vi "RT Main.vi"() -> ()   [LabVIEW 2019]
doc: "The myRIO Custom FPGA Project template acquires button data from the onboard button and displays the button value on a Boolean indicator. The SYS.RDY indicator shows the FPGA status."
uses:
  <vilib>/Platform/TimedLoop/XDataNode/timing_clust.ctl
  <vilib>/Platform/TimedLoop/XDataNode/nitl_modes.ctl
  <vilib>/Platform/TimedLoop/XDataNode/wakeup.ctl
  <vilib>/myRIO/Instrument Drivers/Onboard IO/DIO/typedefs/DIO Reference.ctl
  <vilib>/myRIO/Common/Instrument Driver Framework/Utilities/typedefs/myRIO Generic Hardware Reference.ctl
  <vilib>/myRIO/Common/Instrument Driver Framework/Utilities/typedefs/Hardware Version Enum.ctl
  <vilib>/myRIO/Common/Instrument Driver Framework/Utilities/typedefs/myRIO v1.0 Reference.ctl
  <vilib>/myRIO/Common/Instrument Driver Framework/Utilities/typedefs/Generic FPGA Reference.ctl
  <vilib>/myRIO/Common/Instrument Driver Framework/myRIO v1.0/DIO/typedefs/DIO Channels List.ctl
  <vilib>/myRIO/Common/Instrument Driver Framework/myRIO v1.0/DIO/typedefs/DIO Channels Enum.ctl
  <vilib>/userDefined/High Color/nirio_resource_hc.ctl
  <vilib>/myRIO/Common/Instrument Driver Framework/myRIO v1.0/Encoder/typedefs/Encoder Signal Mode.ctl
  <vilib>/myRIO/Instrument Drivers/Onboard IO/Encoder/typedefs/Encoder Reference.ctl
  <vilib>/myRIO/Common/Instrument Driver Framework/myRIO v1.0/Encoder/typedefs/Encoder Channels Enum.ctl
  <vilib>/myRIO/Common/Instrument Driver Framework/myRIO v1.0/Encoder/typedefs/Encoder Configuration v1.0.ctl
  <vilib>/myRIO/Instrument Drivers/Onboard IO/AO/typedefs/AO Reference.ctl
  <vilib>/myRIO/Common/Instrument Driver Framework/myRIO v1.0/AO/typedefs/AO Channels List.ctl
  <vilib>/myRIO/Common/Instrument Driver Framework/myRIO v1.0/AO/typedefs/AO Channels Enum.ctl
  <vilib>/myRIO/Common/Instrument Driver Framework/Utilities/typedefs/Analog Scaling Constants List.ctl
  <vilib>/myRIO/Common/Instrument Driver Framework/Utilities/typedefs/Analog Scaling Constants.ctl
  <vilib>/myRIO/Common/Instrument Driver Framework/Utilities/vis/Is FPGA Ref Available.vi
  <vilib>/myRIO/Common/Instrument Driver Framework/myRIO v1.0/DIO/vis/myRIO v1.1 Open DIO.vi
  <vilib>/myRIO/Instrument Drivers/Onboard IO/DIO/vis/Read.vi
  <vilib>/myRIO/Instrument Drivers/Onboard IO/DIO/vis/Write.vi
  <vilib>/myRIO/Common/Instrument Driver Framework/myRIO v1.0/Encoder/vis/myRIO v1.1 Open Encoder.vi
  <vilib>/myRIO/Instrument Drivers/Onboard IO/Encoder/vis/Read.vi
  <vilib>/myRIO/Common/Instrument Driver Framework/myRIO v1.0/AO/vis/myRIO v1.1 Open AO.vi
  <vilib>/myRIO/Instrument Drivers/Onboard IO/AO/vis/Write.vi
  <vilib>/myRIO/Common/Instrument Driver Framework/Utilities/vis/Validate Channels.vi
  <vilib>/myRIO/Common/Instrument Driver Framework/myRIO v1.0/DIO/vis/myRIO v1.0 Reserve DIO.vi
  <vilib>/myRIO/Common/Instrument Driver Framework/myRIO v1.0/Encoder/vis/myRIO v1.0 Reserve Encoder.vi
  <vilib>/myRIO/Common/Instrument Driver Framework/myRIO v1.0/AO/vis/myRIO v1.0 Reserve AO.vi
  <vilib>/myRIO/Common/Instrument Driver Framework/myRIO v1.0/Resource Manager/vis/myRIO v1.0 Reserve Channel List.vi
  <vilib>/myRIO/Common/Instrument Driver Framework/myRIO v1.0/DIO/vis/myRIO v1.0 Build MUX Configuration DIO.vi
  <vilib>/myRIO/Common/Instrument Driver Framework/myRIO v1.0/Encoder/vis/myRIO v1.0 Build MUX Configuration Encoder.vi
  <vilib>/myRIO/Common/Instrument Driver Framework/myRIO v1.0/AO/vis/myRIO v1.0 Build MUX Configuration AO.vi
  <vilib>/myRIO/Common/Instrument Driver Framework/myRIO v1.0/Resource Manager/vis/myRIO v1.0 Reserve Channel.vi
  <vilib>/myRIO/Common/Instrument Driver Framework/myRIO v1.0/Resource Manager/vis/myRIO v1.0 Unreserve Channel.vi
  <vilib>/myRIO/Common/Instrument Driver Framework/myRIO v1.0/Resource Manager/vis/myRIO v1.0 Create Configuration List.vi
  <vilib>/myRIO/Common/Instrument Driver Framework/myRIO v1.0/Resource Manager/vis/myRIO v1.0 Build Mutex Name.vi
  <vilib>/FPGAPlugInAG/myRIO-1900/niLvFpga_Open_myRIO-1900.vi
  <vilib>/rvi/interface/common/dynamic/niFpgaDynamicAddResources.vi
  <vilib>/myRIO/Common/Instrument Driver Framework/Utilities/vis/FPGA Ref Manager.vi
  <vilib>/Utility/error.llb/Error Cluster From Error Code.vi
  <vilib>/myRIO/Common/Instrument Driver Framework/Utilities/vis/Ref Counter.vi
  <vilib>/Utility/VariantDataType/GetNumericInfo.vi
  <vilib>/myRIO/Common/Instrument Driver Framework/myRIO v1.0/myRIO v1.1 Open.vi
  <vilib>/myRIO/Common/Instrument Driver Framework/Utilities/vis/IO Manager.vi
  <vilib>/myRIO/Common/Instrument Driver Framework/Utilities/vis/Configuration Manager.vi
  <vilib>/myRIO/Common/Instrument Driver Framework/myRIO v1.0/Resource Manager/vis/myRIO v1.0 Configure IO.vi
  <vilib>/myRIO/Common/Instrument Driver Framework/myRIO v1.0/myRIO v1.0 Close.vi
  <vilib>/myRIO/Common/Instrument Driver Framework/myRIO v1.0/DIO/vis/myRIO v1.0 Read DIO.vi
  <vilib>/myRIO/Common/Instrument Driver Framework/myRIO v1.0/DIO/vis/myRIO v1.0 Write DIO.vi
  <vilib>/myRIO/Common/Instrument Driver Framework/myRIO v1.0/Encoder/vis/myRIO v1.0 Configure Encoder.vi
  <vilib>/myRIO/Common/Instrument Driver Framework/myRIO v1.0/Encoder/vis/myRIO v1.0 Read Encoder.vi
  <vilib>/myRIO/Common/Instrument Driver Framework/myRIO v1.0/AO/vis/myRIO v1.0 Get Scaling Constants AO.vi
  <vilib>/myRIO/Common/Instrument Driver Framework/myRIO v1.0/AO/vis/myRIO v1.0 Write AO.vi
  <vilib>/FPGAPlugInAG/Dynamic/niLvFpga_Close_Dynamic.vi
  <vilib>/rvi/interface/nirviOpenFPGA/nirviOpenFPGA.xnode
  FPGA Bitfiles/hapticdevice2dof_FPGATarget_FPGAMainDefault_0mKZiwDuvEs.lvbitx
  FPGA Main Default.vi
  <vilib>/Platform/TimedLoop/XDataNode/XDataNode.xnode
  <vilib>/myRIO/Express VI/Onboard Devices/Button/Button Express VI.xnode
  <vilib>/myRIO/Instrument Drivers/Onboard IO/DIO/vis/myRIO DIO Open.xnode
  <vilib>/myRIO/Express VI/Onboard IO/DI/DI Express VI.xnode
  <vilib>/myRIO/Express VI/Onboard Devices/LED/LED Express VI.xnode
  <vilib>/myRIO/Express VI/Onboard IO/Encoder/Encoder Express VI.xnode
  <vilib>/myRIO/Instrument Drivers/Onboard IO/Encoder/vis/myRIO Encoder Open.xnode
  <vilib>/myRIO/Common/Instrument Driver Framework/myRIO v1.0/Encoder/typedefs/Encoder Count Direction Enum.ctl
  <vilib>/myRIO/Express VI/Onboard IO/DO/DO Express VI.xnode
  <vilib>/myRIO/Express VI/Onboard IO/AO/AO Express VI.xnode
  <vilib>/myRIO/Instrument Drivers/Onboard IO/AO/vis/myRIO AO Open.xnode
  <vilib>/rvi/interface/nirviCloseFPGA/nirviCloseFPGA.xnode
  <vilib>/myRIO/Instrument Drivers/Utilities/Utilities.lvlib
  <vilib>/Platform/TimedLoop/XDataNode/XDNodeRunTimeDep.lvlib
  <vilib>/myRIO/Instrument Drivers/Onboard IO/Encoder/Encoder.lvlib
  <vilib>/myRIO/Instrument Drivers/Onboard IO/DIO/DIO.lvlib
  <vilib>/myRIO/Instrument Drivers/Onboard IO/AO/AO.lvlib
panel:
  in  "Ctrl Hz":i64=1000
  in  "TX Hz":i64=1000
  in  "RX Hz":i64=1000
  out "Encoder Reset":bool
  out "Controller\nFinished Late":bool
  out "UDP Read\nFinished Late":bool
  out "UDP Write\nFinished Late":bool
  out "Index":bool
  in  "Current Limit":dbl=1.0
  out "UDP":bool
  out "y_0":dbl
  out "x_0":dbl
  out "STOP":bool
  out "Status":i32
  out "F_y":dbl
  out "F_x":dbl
  in  "?":bool
  in  "Direction A":bool
  in  "Direction B":bool
  in  "Current A":dbl(slide) scale=0.0..10.0
  in  "Current B":dbl(slide) scale=0.0..10.0
  in  "switch":bool=TRUE
  in  "Enable":bool=TRUE
  out "I_0":dbl format="%#.2g"
  out "I_1":dbl format="%#.2g"
  out "f_x":dbl
  out "f_y":dbl
  out "x":dbl format="%#.2g"
  out "y":dbl format="%#.2g"
  out "XY 그래프":cluster{dbl[], dbl[]}(graph)={[-0.04564152437153268], [-0.14073615837554598]}
  out "y_dot":dbl
  out "x_dot":dbl
  in  "Stiff":dbl=1.0
  in  "Damp":dbl
  out "Counter A":i32
  out "Counter B":i32
  out "ENC A":ext
  out "ENC B":ext
  out "count":ext format="%-#.3g"
  out "miss":u32
  out "error out":errorcluster
  # "Manual Control"
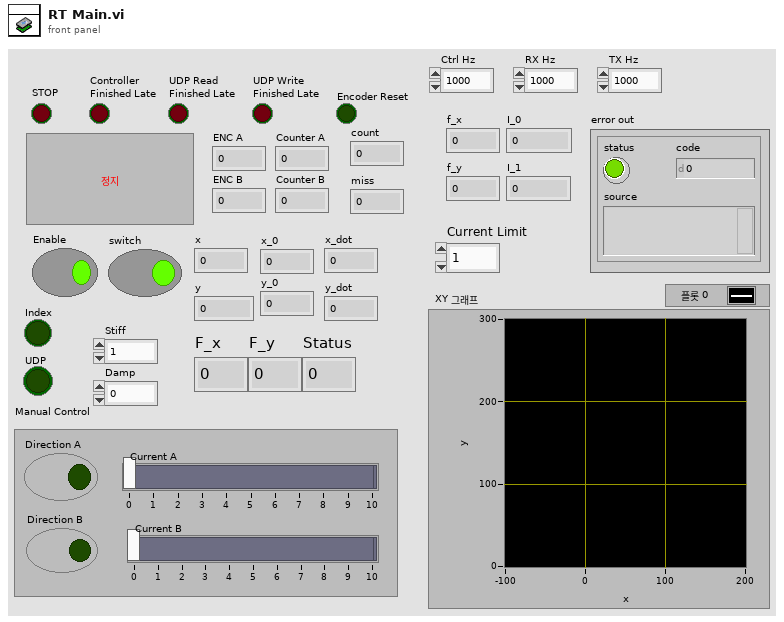
[diagram p1: front panel]
types:
  T1 = typedef "DIO.lvlib/DIO Reference.ctl" = cluster{"myRIO Reference":T2, "DIO Channels List":T6}
  T2 = typedef "myRIO Generic Hardware Reference.ctl" = cluster{"myRIO Model":T3, "myRIO Hardware Reference":T4}
  T3 = typedef "Hardware Version Enum.ctl" = enum16{"Unknown", "myRIO-1900", "myRIO-1950", "roboRIO", "NI ELVIS RIO CM", "ELVIS III"}
  T4 = typedef "myRIO v1.0 Reference.ctl" = cluster{"Generic FPGA Reference":T5, "Allow multiple opens":bool}
  T5 = typedef "Generic FPGA Reference.ctl" = refnum<k20>
  T6 = typedef "DIO Channels List.ctl" = T7[]
  T7 = typedef "DIO Channels Enum.ctl" = enum16{"Not Connected", "C/DIO0", "C/DIO1", "C/DIO2", "C/DIO3", "C/DIO4", "C/DIO5", "C/DIO6", "C/DIO7", "A/DIO0", "A/DIO1", "A/DIO2", "A/DIO3", "A/DIO4", "A/DIO5", "A/DIO6", "A/DIO7", "A/DIO8", "A/DIO9", "A/DIO10", "A/DIO11", "A/DIO12", "A/DIO13", "A/DIO14", "A/DIO15", "A/DIO16", "A/DIO17", "A/DIO18", "A/DIO19", "B/DIO0", "B/DIO1", "B/DIO2", "B/DIO3", "B/DIO4", "B/DIO5", "B/DIO6", "B/DIO7", "B/DIO8", "B/DIO9", "B/DIO10", "B/DIO11", "B/DIO12", "B/DIO13", "B/DIO14", "B/DIO15", "B/DIO16", "B/DIO17", "B/DIO18", "B/DIO19", "LED0", "LED1", "LED2", "LED3", "Button0", "DIO/DIO0", "DIO/DIO1", "DIO/DIO2", "DIO/DIO3", "DIO/DIO4", "DIO/DIO5", "DIO/DIO6", "DIO/DIO7", "DIO/DIO8", "DIO/DIO9", "SPI/CS0", "SPI/CS1", "SPI/CS2", "SPI/CS3", "LED RADIO (Green)", "LED RADIO (Red)", "LED COMM (Green)", "LED COMM (Red)", "LED MODE (Green)", "LED MODE (Red)"}
  T8 = typedef "nirio_resource_hc.ctl" = tag
  T9 = typedef "XDNodeRunTimeDep.lvlib/timing_clust.ctl" = cluster{"Expected End [f-1]":u64, "Actual End [f-1]":u64, "Finished Late? [f-1]":bool, "Expected End [i-1]":u64, "Actual End [i-1]":u64, "Finished Late? [i-1]":bool, "Expected Start [i]":u64, "Actual Start [i]":u64, "Expected Start [f]":u64, "Actual Start [f]":u64, "Source Name":string, "Structure Name":string, "Period":i64, "Deadline":i64, "Offset":i64, "Start":i64, "Priority":i32, "Timeout":i32, "Mode":T10, "Wakeup Reason":T11, "Error":errorcluster, "Source Type":string, "Secondary Source Type":string, "Global End Time":u64, "Global Start Time":u64, "Frame Duration":u64, "Iteration Duration":u64, "Assigned CPU":i32, "I/O Scan Engine Mode":u32}
  T10 = typedef "XDNodeRunTimeDep.lvlib/nitl_modes.ctl" = enum32{"No Change", "Process missed periods, maintain original phase", "Discard missed periods, maintain original phase", "Process missed periods, ignore original phase", "Discard missed periods, ignore original phase"}
  T11 = typedef "XDNodeRunTimeDep.lvlib/wakeup.ctl" = enum32{"Normal", "Aborted", "Asynchronous wakeup", "Timing source error", "Timed loop error", "Timeout"}
  T12 = typedef "Encoder.lvlib/Encoder Reference.ctl" = cluster{"myRIO Reference":T2, "Encoder Channels Enum":T13}
  T13 = typedef "Encoder Channels Enum.ctl" = enum16{"Not Connected", "C/ENC0", "C/ENC1", "A/ENC", "A/ENC0", "A/ENC1", "A/ENC2", "A/ENC3", "A/ENC4", "A/ENC5", "A/ENC6", "A/ENC7", "A/ENC8", "A/ENC9", "B/ENC", "B/ENC0", "B/ENC1", "B/ENC2", "B/ENC3", "B/ENC4", "B/ENC5", "B/ENC6", "B/ENC7", "B/ENC8", "B/ENC9", "DIO/ENC0", "DIO/ENC1", "DIO/ENC2", "DIO/ENC3", "DIO/ENC4"}
  T14 = typedef "Encoder Signal Mode.ctl" = enum16{"Quadrature phase signal", "Step and direction signal"}
  T15 = typedef "AO.lvlib/AO Reference.ctl" = cluster{"myRIO Reference":T2, "AO Channel List":T16, "AO Scaling Constant List":T18}
  T16 = typedef "AO Channels List.ctl" = T17[]
  T17 = typedef "AO Channels Enum.ctl" = enum16{"Not Connected", "AudioOut/Left", "AudioOut/Right", "C/AO0", "C/AO1", "A/AO0", "A/AO1", "B/AO0", "B/AO1"}
  T18 = typedef "Analog Scaling Constants List.ctl" = T19[]
  T19 = typedef "Analog Scaling Constants.ctl" = cluster{"LSB Weight (Volts)":dbl, "Offset (Volts)":dbl, "Signed?":bool}
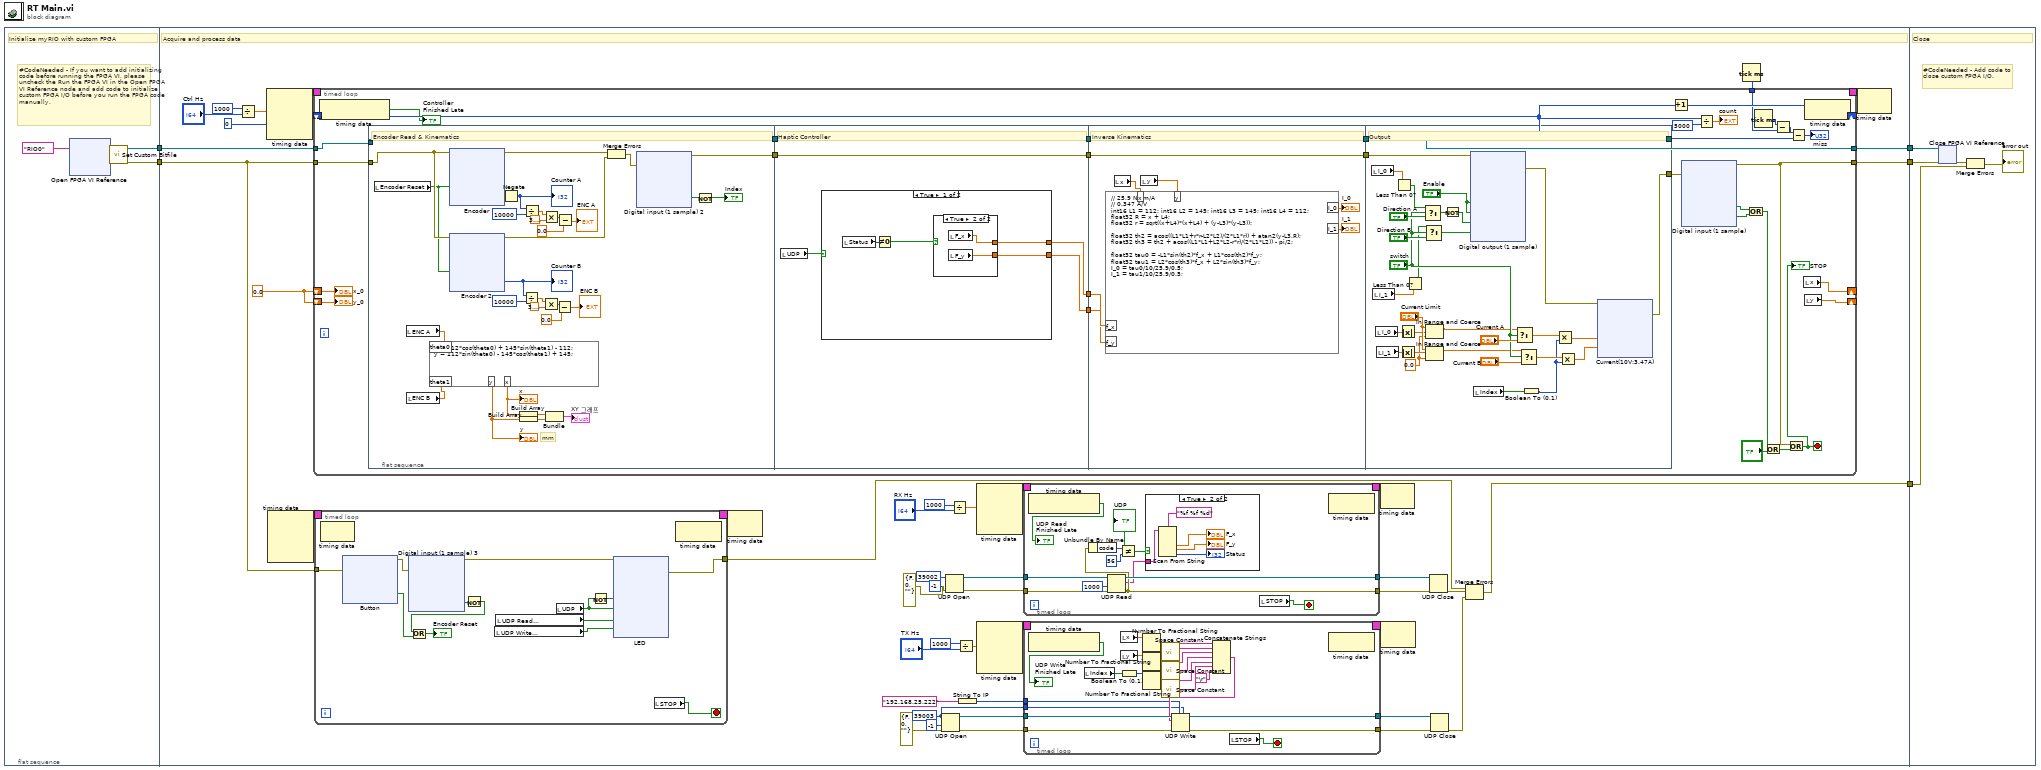
[diagram p0: block diagram]
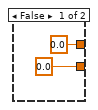
[diagram p3: hidden frame]
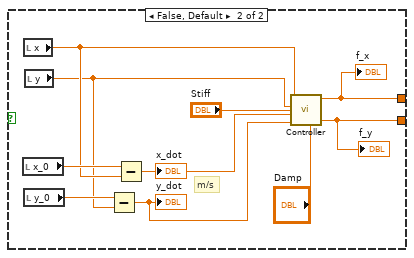
[diagram p4: hidden frame]
diagram:
  n1 = flat-sequence {
    tunnel: [w6] -> w5
    tunnel: [w7] -> w4
    tunnel: w5 -> [w21]
    tunnel: w4 -> [w22]
    tunnel: [w49] -> w3
    tunnel: [w48] -> w2
    tunnel: [w25] -> w1
    tunnel: w3 -> [w605]
    tunnel: w2 -> [w604]
    tunnel: w1 -> [w601]
    frame #0 {
      # "#CodeNeeded - If you want to add initializing code before running the FPGA VI, please uncheck the Run the FPGA VI in the Open FPGA VI Reference node and add code to initialize custom FPGA I/O before you run the FPGA code manually."
      # "Initialize myRIO with custom FPGA"
      n2 = xnode "Open FPGA VI Reference"("resource name"=tag "RIO0") -> ("FPGA VI Reference Out"=w8:refnum<k20>, "error out"=w9:errorcluster)  [unwired: 1 in]
      n3 = call <vilib>:"Set Custom Bitfile.vi"("error in (no error)"=w9, "Custom FPGA Reference In"=w8) -> ("error out"=w6:errorcluster, "Custom FPGA Reference Out"=w7:refnum<k20>)  [unwired: 8 in]
    }
    frame #1 {
      w28 = u16 39003 ("port")
      w51 = 0.0
      # "Acquire and process data"
      n4 = Divide(x=i64 1000, y="Ctrl Hz") -> (x/y=w11:dbl)
      n5 = node-c288(w11) -> (w54:T9)  [unwired: 3 in]
      n6 = node-c288() -> (w24:T9)  [unwired: 4 in]
      n7 = timed-loop {
        timing: w24 -> [_]
        timing-out: [_] -> w23
        tunnel: w21 -> [w67]
        tunnel: [w66] -> w20
        stop <- w61 stop-if-true
        n8 = node-c288() -> ()  [unwired: 1 in, 1 out]
        n9 = xnode "Button"("error in (no error)"=w67) -> ("Value"=w56:bool, "error out"=w60:errorcluster)
        n10 = xnode "Digital input (1 sample) 3"("error in (no error)"=w60) -> ("Encoder Reset (A/DIO5 (Pin 21))"=w58:bool, "error out"=w59:errorcluster)
        n11 = Not(x=w58) -> (.not. x?=w55:bool)
        n12 = Or(x=w55, y=w56) -> (x .or. y?=→"Encoder Reset":bool)
        n13 = local read "UDP Write\nFinished Late"() -> (w62:bool)
        n14 = local read "UDP Read\nFinished Late"() -> (w63:bool)
        n15 = local read "UDP"() -> (w64:bool)
        n16 = Not(x=w64) -> (.not. x?=w65:bool)
        n17 = xnode "LED"("Local Mode"=w65, "UDP Mode"=w64, "UDP Read Error"=w63, "UDP Write Error"=w62, "error in (no error)"=w59) -> ("error out"=w66:errorcluster)
        n18 = local read "STOP"() -> (w61:bool)
        n19 = node-c288() -> ()  [unwired: 1 in, 1 out]
      }
      n20 = node-c288(w23) -> ()  [unwired: 1 out]
      n21 = UDP Open(8:errorcluster {"status"=FALSE, "code"=0, "source"=""} ("error in (no error)"), 9:-1 ("timeout ms (25000)"), 11:w28) -> (port=w26:refnum<k16>, 0:w27:errorcluster)  [unwired: 2 in, 1 out]
      n22 = UDP Open(8:errorcluster {"status"=FALSE, "code"=0, "source"=""} ("error in (no error)"), 9:-1 ("timeout ms (25000)"), 11:u16 39002 ("port")) -> (port=w33:refnum<k16>, 0:w34:errorcluster)  [unwired: 2 in, 1 out]
      n23 = Divide(x=i64 1000, y="RX Hz") -> (x/y=w17:dbl)
      n24 = Divide(x=i64 1000, y="TX Hz") -> (x/y=w14:dbl)
      n25 = String To IP(1:"192.168.25.222" ("이름")) -> (0:w29:u32)
      n26 = node-c288(w17) -> (w47:T9)  [unwired: 3 in]
      n27 = node-c288(w14) -> (w45:T9)  [unwired: 3 in]
      n28 = timed-loop {
        timing: w47 -> [_]
        timing-out: [_] -> w46
        tunnel: w33 -> [w216]
        tunnel: w34 -> [w217]
        tunnel: [w214] -> w41
        tunnel: [w211] -> w40
        stop <- w208 stop-if-true
        n29 = node-c288() -> (→"UDP Read\nFinished Late":bool)  [unwired: 1 in]
        n30 = UDP Read(connection ID=w216, timeout ms (25000)=1000, 8:w217) -> (data out=w209:string, error out=w211:errorcluster, 3:w214:refnum<k16>)  [unwired: 1 in, 2 out]
        n31 = Unbundle By Name(w211) -> ("code"=w213:i32)
        n32 = Not Equal?(x=w213, y=56) -> (x != y?=w210:bool)
        "UDP" <- w210
        n33 = case shown="True" w210 {
          tunnel: w209 -> [_ w222]
          frame False {
          }
          frame True {
            n34 = Scan From String(format string="%f %f %d", input string=w222) -> (output 1=→"F_x":dbl, output 2=→"F_y":dbl, output 3=→"Status":i32)  [unwired: 5 in, 3 out]
          }
        }
        n35 = local read "STOP"() -> (w208:bool)
        n36 = node-c288() -> ()  [unwired: 1 in, 1 out]
      }
      n37 = timed-loop {
        timing: w45 -> [_]
        timing-out: [_] -> w44
        tunnel: w26 -> [w198]
        tunnel: w27 -> [w199]
        tunnel: w29 -> [w190]
        tunnel: w28 -> [w189]
        tunnel: [w188] -> w43
        tunnel: [w187] -> w42
        stop <- w182 stop-if-true
        n38 = node-c288() -> (→"UDP Write\nFinished Late":bool)  [unwired: 1 in]
        n39 = local read "Index"() -> (w180:bool)
        n40 = local read "x"() -> (w197:dbl)
        n41 = local read "y"() -> (w194:dbl)
        n42 = Boolean To (0,1)(Boolean=w180) -> (0, 1=w183:i16)
        n43 = Number To Fractional String(number=w197) -> (F-format string=w196:string)  [unwired: 3 in]
        n44 = Number To Fractional String(number=w194) -> (F-format string=w193:string)  [unwired: 3 in]
        n45 = Number To Fractional String(number=w183) -> (F-format string=w186:string)  [unwired: 3 in]
        n46 = call <vilib>:"Space Constant.vi"() -> ("String"=w195:string)
        n47 = call <vilib>:"Space Constant.vi"() -> ("String"=w192:string)
        n48 = call <vilib>:"Space Constant.vi"() -> ("String"=w185:string)
        n49 = Concatenate Strings(w196, w195, w193, w192, w186, w185, "\r") -> (w191:string)
        n50 = UDP Write(address=w190, port or service name=w189, connection ID=w198, data in=w191, 8:w199) -> (error out=w187:errorcluster, 3:w188:refnum<k16>)  [unwired: 1 in]
        n51 = local read "STOP"() -> (w182:bool)
        n52 = node-c288() -> ()  [unwired: 1 in, 1 out]
      }
      n53 = node-c288(w46) -> ()  [unwired: 1 out]
      n54 = node-c288(w44) -> ()  [unwired: 1 out]
      n55 = UDP Close(connection ID=w41, 8:w40) -> (error out=w39:errorcluster)  [unwired: 1 out]
      n56 = UDP Close(connection ID=w43, 8:w42) -> (error out=w38:errorcluster)  [unwired: 1 out]
      n57 = Merge Errors(w20, w39, w38) -> (w25:errorcluster)
      n58 = Tick Count (ms)() -> (millisecond timer value=w50:u32)
      n59 = timed-loop {
        timing: w54 -> [_]
        timing-out: [_] -> w53
        tunnel: w22 -> [w259]
        tunnel: [w260] -> w49
        tunnel: w21 -> [w261]
        tunnel: [w247] -> w48
        shift-right: [w254] -> _
        shift-left: u32 0 -> [w249]
        shift-right: [w238] -> _
        shift-left: w51 -> [w240]
        shift-right: [w237] -> _
        shift-left: w51 -> [w239]
        tunnel: w50 -> [w252]
        stop <- w233 stop-if-true
        n60 = node-c288() -> (→"Controller\nFinished Late":bool)  [unwired: 1 in]
        n61 = flat-sequence {
          tunnel: w261 -> [w300]
          tunnel: [w302] -> w231
          tunnel: w259 -> [w325]
          tunnel: [w325] -> w232
          tunnel: [w460] -> w244
          tunnel: [w459] -> w243
          tunnel: [w458] -> w242
          tunnel: [w457] -> w241
          tunnel: w232 -> [w459]
          tunnel: w231 -> [w460]
          tunnel: w244 -> [w486]
          tunnel: [w486] -> w258
          tunnel: w243 -> [w485]
          tunnel: [w485] -> w257
          tunnel: w242 -> [w482]
          tunnel: w241 -> [w481]
          tunnel: [w502] -> w246
          tunnel: w258 -> [w512]
          tunnel: [w511] -> w260
          tunnel: w257 -> [w511]
          frame #0 {
            # "mm"
            # "Encoder Read & Kinematics"
            n62 = local read "Encoder Reset"() -> (w299:bool)
            n63 = local read "ENC A"() -> (w308:ext)
            n64 = local read "ENC B"() -> (w309:ext)
            n65 = formula code="x = 112*cos(theta0) + 145*sin(theta1) - 112;\ny = 112*sin(theta0) - 145*cos(theta1) + 145;"("theta0"=w308, "theta1"=w309) -> ("x"=w312:dbl, "y"=w307:dbl)
            "x" <- w312
            "y" <- w307
            n66 = xnode "Encoder"("Reset Counter"=w299, "error in (no error)"=w300) -> ("Counter Value"=w323:i32, "error out"=w328:errorcluster)  [unwired: 2 out]
            n67 = xnode "Encoder 2"("Reset Counter"=w299, "error in (no error)"=w300) -> ("Counter Value"=w315:i32, "error out"=w327:errorcluster)  [unwired: 2 out]
            "Counter B" <- w315
            n68 = Negate(x=w323) -> (-x=w313:i32)
            "Counter A" <- w313
            n69 = Build Array(w312) -> (w311:dbl[])
            n70 = Build Array(w307) -> (w310:dbl[])
            n71 = Divide(x=w315, y=10000) -> (x/y=w318:dbl)
            n72 = Divide(x=w313, y=10000) -> (x/y=w322:dbl)
            n73 = Multiply(x=w318, y=3.141592653589793) -> (x*y=w319:dbl)
            n74 = Multiply(x=w322, y=3.141592653589793) -> (x*y=w326:dbl)
            n75 = Bundle(w311, w310) -> (→"XY 그래프":cluster{dbl[], dbl[]})  [unwired: 1 in]
            n76 = Subtract(x=w319, y=0.0) -> (x-y=→"ENC B":dbl)
            n77 = Subtract(x=w326, y=0.0) -> (x-y=→"ENC A":dbl)
            n78 = Merge Errors(w328, w327) -> (w303:errorcluster)
            n79 = xnode "Digital input (1 sample) 2"("error in (no error)"=w303) -> ("Index (A/DIO3 (Pin 17))"=w301:bool, "error out"=w302:errorcluster)
            n80 = Not(x=w301) -> (.not. x?=→"Index":bool)
          }
          frame #1 {
            # "Haptic Controller"
            n81 = local read "UDP"() -> (w456:bool)
            n82 = case shown="True" w456 {
              tunnel: [w464 w474] -> w458
              tunnel: [w463 w473] -> w457
              frame True {
                n83 = local read "Status"() -> (w461:i32)
                n84 = Not Equal To 0?(x=w461) -> (x != 0?=w462:bool)
                n85 = case shown="True" w462 {
                  tunnel: [0.0 ("F_x") w468] -> w464
                  tunnel: [0.0 ("F_y") w467] -> w463
                  frame False {
                  }
                  frame True {
                    n86 = local read "F_x"() -> (w468:dbl)
                    n87 = local read "F_y"() -> (w467:dbl)
                  }
                }
              }
              frame False, Default {
                # "m/s"
                n88 = local read "x_0"() -> (w472:dbl)
                n89 = local read "x"() -> (w470:dbl)
                n90 = local read "y_0"() -> (w471:dbl)
                n91 = local read "y"() -> (w469:dbl)
                n92 = Subtract(x=w471, y=w469) -> (x-y=w478:dbl)
                "y_dot" <- w478
                n93 = Subtract(x=w472, y=w470) -> (x-y=w477:dbl)
                "x_dot" <- w477
                n94 = call "Controller.vi"("x"=w470, "y"=w469, "x_dot"=w477, "y_dot"=w478, "Stiff"="Stiff", "Damp"="Damp") -> ("f_x"=w474:dbl, "f_y"=w473:dbl)  [unwired: 3 in]
                "f_x" <- w474
                "f_y" <- w473
              }
            }
          }
          frame #2 {
            # "Inverse Kinematics"
            n95 = local read "x"() -> (w480:dbl)
            n96 = local read "y"() -> (w479:dbl)
            n97 = formula code="// 25.9 Nmm/A\n// 0.347 A/V\nint16 L1 = 112; int16 L2 = 145; int16 L3 = 145; int16 L4 = 112;\nfloat32 R = x + L4;\nfloat32 r = sqrt((x+L4)*(x+L4) + (y-L3)*(y-L3));\n\nfloat32 th2 = acos((L1*L1+r*r-L2*L2)/(2*L1*r)) + atan2(y-L3,R);\nfloat32 th3 = th2 + acos((L1*L1+L2*L2-r*r)/(2*L1*L2)) - pi/2;\n\nfloat32 tau0 = -L1*sin(th2)*f_x + L1*cos(th2)*f_y;\nfloat32 tau1 = L2*cos(th3)*f_x + L2*sin(th3)*f_y;\nI_0 = tau0/10/25.9/0.5;\nI_1 = tau1/10/25.9/0.5;"("f_x"=w482, "f_y"=w481, "x"=w480, "y"=w479) -> ("I_0"=→"I_0":dbl, "I_1"=→"I_1":dbl)
          }
          frame #3 {
            w493 = 0.0 ("lower limit")
            # "Output"
            n98 = local read "I_0"() -> (w506:dbl)
            n99 = local read "I_1"() -> (w504:dbl)
            n100 = local read "I_0"() -> (w516:dbl)
            n101 = local read "I_1"() -> (w517:dbl)
            n102 = Less Than 0?(x=w506) -> (x < 0?=w505:bool)
            n103 = Absolute Value(x=w516) -> (abs(x)=w497:dbl)
            n104 = Absolute Value(x=w517) -> (abs(x)=w496:dbl)
            n105 = Less Than 0?(x=w504) -> (x < 0?=w503:bool)
            n106 = Select(t=w505, s="switch", f="Direction A") -> (s? t:f=w509:bool)
            n107 = Select(t=w503, s="switch", f="Direction B") -> (s? t:f=w499:bool)
            n108 = In Range and Coerce(upper limit="Current Limit", x=w497, lower limit=w493) -> (coerced(x)=w494:dbl)  [unwired: 1 out]
            n109 = In Range and Coerce(upper limit="Current Limit", x=w496, lower limit=w493) -> (coerced(x)=w495:dbl)  [unwired: 1 out]
            n110 = Not(x=w509) -> (.not. x?=w500:bool)
            n111 = xnode "Digital output (1 sample)"("Enable A (A/DIO0 (Pin 11))"="Enable", "Enable B (B/DIO0 (Pin 11))"="Enable", "Direction A (A/DIO1 (Pin 13))"=w500, "Direction B (B/DIO1 (Pin 13))"=w499, "error in (no error)"=w512) -> ("error out"=w513:errorcluster)
            n112 = local read "Index"() -> (w488:bool)
            n113 = Select(t=w494, s="switch", f="Current A") -> (s? t:f=w492:dbl)
            n114 = Select(t=w495, s="switch", f="Current B") -> (s? t:f=w490:dbl)
            n115 = Boolean To (0,1)(Boolean=w488) -> (0, 1=w487:i16)
            n116 = Multiply(x=w492, y=w487) -> (x*y=w491:dbl)
            n117 = Multiply(x=w490, y=w487) -> (x*y=w489:dbl)
            n118 = xnode "Current(10V:3.47A)"("Current A (A/AO0 (Pin 2))"=w491, "Current B (B/AO0 (Pin 2))"=w489, "error in (no error)"=w513) -> ("error out"=w502:errorcluster)
          }
        }
        n119 = Increment(x=w249) -> (x+1=w254:u32)
        n120 = xnode "Digital input (1 sample)"("error in (no error)"=w246) -> ("velLimit0 (A/DIO2 (Pin 15))"=w235:bool, "velLimit1 (B/DIO2 (Pin 15))"=w234:bool, "error out"=w247:errorcluster)
        n121 = Divide(x=w249, y=u16 5000) -> (x/y=→"count":dbl)
        n122 = Or(x=w235, y=w234) -> (x .or. y?=w236:bool)
        n123 = Tick Count (ms)() -> (millisecond timer value=w253:u32)
        n124 = Or(x=w236, y="?") -> (x .or. y?=w248:bool)
        n125 = Subtract(x=w253, y=w252) -> (x-y=w251:u32)
        n126 = Or(x=w247, y=w248) -> (x .or. y?=w233:bool)
        "STOP" <- w233
        n127 = Subtract(x=w251, y=w249) -> (x-y=→"miss":u32)
        n128 = local read "x"() -> (w238:dbl)
        n129 = local read "y"() -> (w237:dbl)
        n130 = node-c288() -> ()  [unwired: 1 in, 1 out]
        "x_0" <- w240
        "y_0" <- w239
      }
      n131 = node-c288(w53) -> ()  [unwired: 1 out]
    }
    frame #2 {
      # "#CodeNeeded - Add code to close custom FPGA I/O."
      # "Close"
      n132 = xnode "Close FPGA VI Reference"("FPGA VI Reference In"=w605, "error in"=w604) -> ("error out"=w603:errorcluster)
      n133 = Merge Errors(w603, w601) -> (→"error out":errorcluster)
    }
  }
